vi "Load.vi"(8 "error in (no error)":errorcluster, 11 "SPXMusicLibrary in":refnum<class "SPXMusicLibrary.lvclass">) -> (0 "error out":errorcluster, 3 "SPXMusicLibrary out":refnum<class "SPXMusicLibrary.lvclass">)   [LabVIEW 2015, in "SPXMusicLibrary.lvclass"]
uses:
  SPXMusicLibrary.lvclass
  MusicLibrary.lvclass
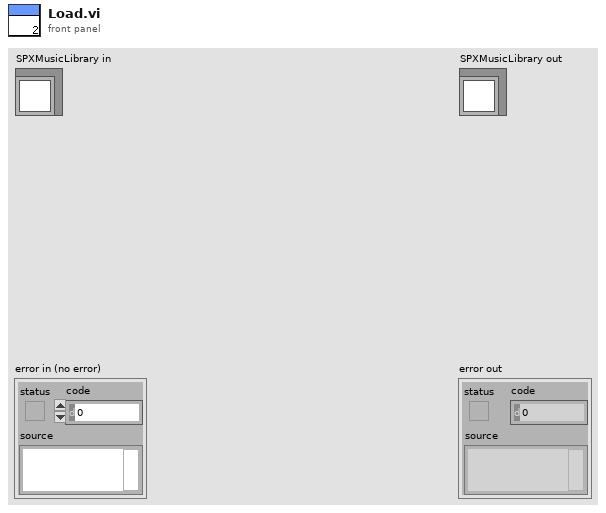
[diagram p1: front panel]
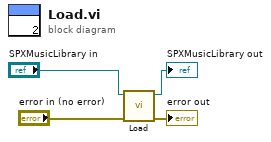
[diagram p0: block diagram]
diagram:
  n1 = call-parent "Load.vi"("error in (no error)"="error in (no error)", "MusicLibrary in"="SPXMusicLibrary in") -> ("error out"=→"error out":errorcluster, "MusicLibrary out"=→"SPXMusicLibrary out":refnum<class "SPXMusicLibrary.lvclass">)  [unwired: 8 in]
